vi "CRYChange post_xyz mode.vi"(6 "Wave In":T2={"Waveform"={"X0"=0.0, "dX"=0.0, "Y"=[]}, "X data"=1, "Y data"=0, "Y axis"=0, "X unit"="s", "Y unit"="", "Y dB ref"=1.0, "display Y"=TRUE, "display X"=FALSE, "Overload?"=FALSE, "Test Info"="", "Step No."=0, "Name"="", "protected"=FALSE, "Sqc history"=[], "Signal Channel ID"=0, "Plot Settings"={"Color"=0, "Interpolation"=0, "Point Style"=0, "Line Style"=0, "Point Color"=0, "Line Width"=0, "Bar Plot Style"=0, "Fill To"=0}, "AutoProtect"=FALSE} {"Y dB ref" format="%.1f"; "Y axis" items=["Log", "Lin"]; "Y data" items=["dB", "Lin"]; "X data" items=["dB", "Lin"]}, 7 "Work in":u16(slide), 8 "Value In":T1={"Name"="", "Curve"=[], "X data"=1, "Y data"=1, "Z data"=1, "X axis"=0, "Y axis"=1, "Z axis"=1, "X unit"="Hz", "Y unit"="", "Z unit"="deg.", "X dB ref"=1.0, "Y dB ref"=1.0, "Z dB ref"=1.0, "single val"=FALSE, "protected"=FALSE, "display X"=TRUE, "display Y"=TRUE, "display Z"=TRUE, "Test Info"="", "Step No."=0, "Plot Settings"={"Color"=0, "Interpolation"=0, "Point Style"=0, "Line Style"=0, "Point Color"=0, "Line Width"=0, "Bar Plot Style"=0, "Fill To"=0}, "AutoProtect"=FALSE} {"Z data" items=["dB", "Lin"]; "X data" items=["dB", "Lin"]; "Y data" items=["dB", "Lin"]; "Z dB ref" format="%.1f"; "Z axis" items=["Log", "Lin"]; "X dB ref" format="%.1f"; "X axis" items=["Log", "Lin"]; "Y axis" items=["Log", "Lin"]; "Y dB ref" format="%.1f"; "Curve"."z" format="%.2f"; "Curve"."y" format="%.2f"; "Curve"."x" format="%.2f"}, 9 "Curve In":T1={"Name"="", "Curve"=[], "X data"=1, "Y data"=1, "Z data"=1, "X axis"=0, "Y axis"=1, "Z axis"=1, "X unit"="Hz", "Y unit"="", "Z unit"="deg.", "X dB ref"=1.0, "Y dB ref"=1.0, "Z dB ref"=1.0, "single val"=FALSE, "protected"=FALSE, "display X"=TRUE, "display Y"=TRUE, "display Z"=TRUE, "Test Info"="", "Step No."=0, "Plot Settings"={"Color"=0, "Interpolation"=0, "Point Style"=0, "Line Style"=0, "Point Color"=0, "Line Width"=0, "Bar Plot Style"=0, "Fill To"=0}, "AutoProtect"=FALSE} {"Z data" items=["dB", "Lin"]; "X data" items=["dB", "Lin"]; "Y data" items=["dB", "Lin"]; "Z dB ref" format="%.1f"; "Z axis" items=["Log", "Lin"]; "X dB ref" format="%.1f"; "X axis" items=["Log", "Lin"]; "Y axis" items=["Log", "Lin"]; "Y dB ref" format="%.1f"; "Curve"."z" format="%.2f"; "Curve"."y" format="%.2f"; "Curve"."x" format="%.2f"}, 10 "XYZ Mode In":u16=1, 11 "Type In":enum16{"Curves", "Values", "Results", "WFM"}(ring)) -> (0 "Value":dbl, 1 "Tip Out":string, 2 "Unit Out":string, 3 "Value Out":string, 4 "Is Val&log":u16)   [LabVIEW 2013]
uses:
  Typedef Control/CRYWaveform Cluster.ctl
  Typedef Control/CRYData Cluster.ctl
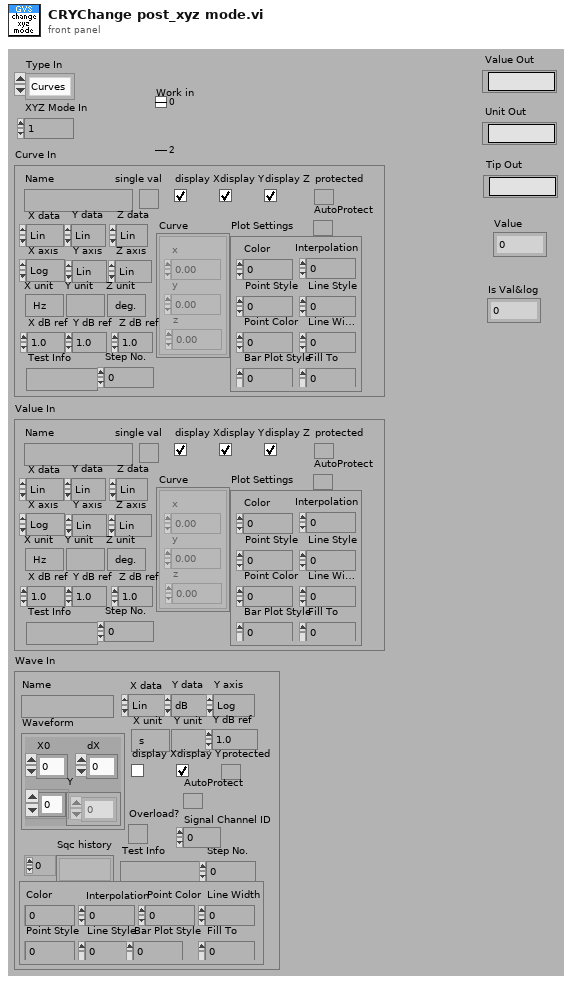
[diagram p1: front panel]
types:
  T1 = typedef "CRYData Cluster.ctl" = cluster{"Name":string, "Curve":cluster{"x":dbl, "y":dbl, "z":dbl}[], "X data":u16, "Y data":u16, "Z data":u16, "X axis":u16, "Y axis":u16, "Z axis":u16, "X unit":string, "Y unit":string, "Z unit":string, "X dB ref":dbl, "Y dB ref":dbl, "Z dB ref":dbl, "single val":bool, "protected":bool, "display X":bool, "display Y":bool, "display Z":bool, "Test Info":string, "Step No.":i32, "Plot Settings":cluster{"Color":u32, "Interpolation":u8, "Point Style":u8, "Line Style":u8, "Point Color":u32, "Line Width":u8, "Bar Plot Style":u8, "Fill To":i16}, "AutoProtect":bool}
  T2 = typedef "CRYWaveform Cluster.ctl" = cluster{"Waveform":cluster{"X0":dbl, "dX":dbl, "Y":sgl[]}, "X data":u16, "Y data":u16, "Y axis":u16, "X unit":string, "Y unit":string, "Y dB ref":dbl, "display Y":bool, "display X":bool, "Overload?":bool, "Test Info":string, "Step No.":i32, "Name":string, "protected":bool, "Sqc history":string[], "Signal Channel ID":i32, "Plot Settings":cluster{"Color":u32, "Interpolation":u8, "Point Style":u8, "Line Style":u8, "Point Color":u32, "Line Width":u8, "Bar Plot Style":u8, "Fill To":i16}, "AutoProtect":bool}
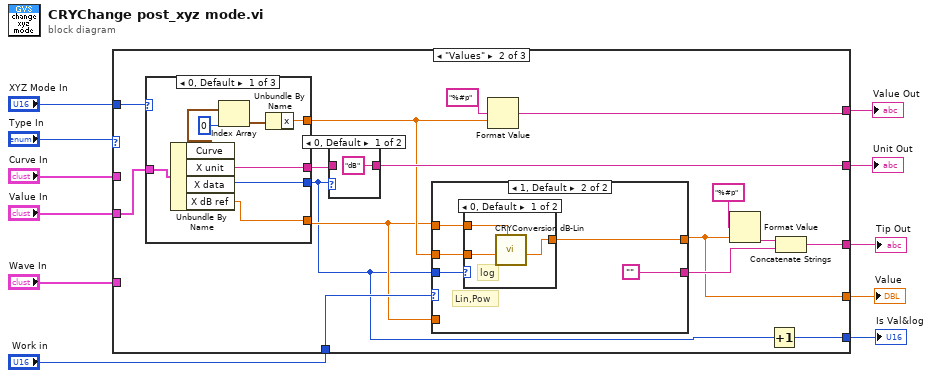
[diagram p0: block diagram]
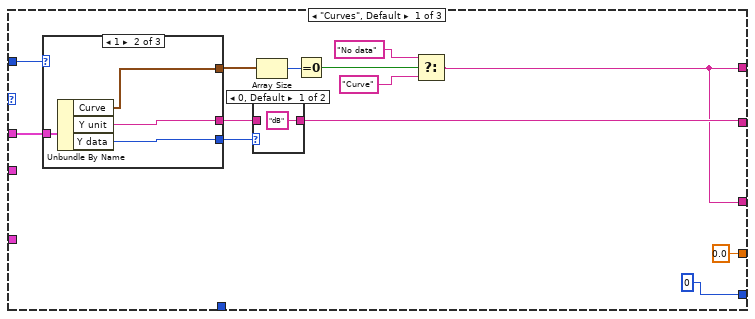
[diagram p2: hidden frame]
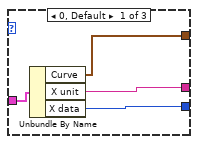
[diagram p4: hidden frame]
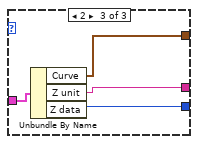
[diagram p5: hidden frame]
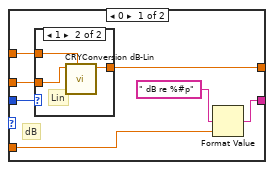
[diagram p7: hidden frame]
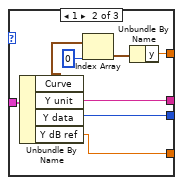
[diagram p10: hidden frame]
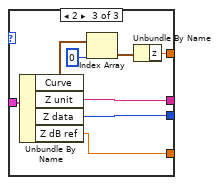
[diagram p11: hidden frame]
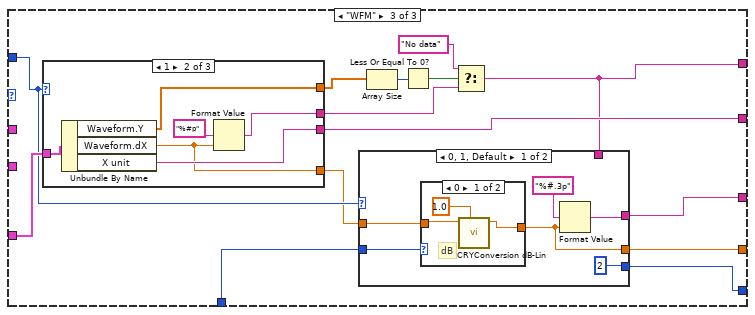
[diagram p12: hidden frame]
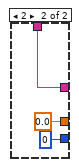
[diagram p14: hidden frame]
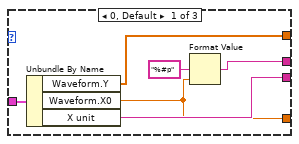
[diagram p15: hidden frame]
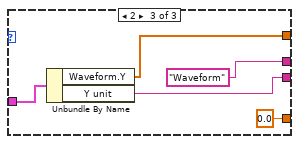
[diagram p16: hidden frame]
diagram:
  n1 = case shown="\"Values\"" "Type In" {
    tunnel: [w20 w48 w114] -> w11
    tunnel: "XYZ Mode In" -> [w24 w54 w107]
    tunnel: "Curve In" -> [w23 _ _]
    tunnel: "Value In" -> [_ w53 _]
    tunnel: "Wave In" -> [_ _ w113]
    tunnel: [w14 w51 w103] -> w4
    tunnel: "Work in" -> [_ w50 w106]
    tunnel: [w14 w44 w104] -> w3
    tunnel: [0.0 ("dX") w41 w102] -> w2
    tunnel: [0 w39 w101] -> w1
    frame "Curves", Default {
      n2 = case shown="1" w24 {
        tunnel: w23 -> [w30 w34 w38]
        tunnel: [w29 w33 w37] -> w21
        tunnel: [w28 w32 w36] -> w22
        tunnel: [w27 w31 w35] -> w18
        frame 0, Default {
          n3 = Unbundle By Name(w30) -> ("Curve"=w27:cluster{"x":dbl, "y":dbl, "z":dbl}[], "X unit"=w29:string, "X data"=w28:u16)
        }
        frame 1 {
          n4 = Unbundle By Name(w34) -> ("Curve"=w31:cluster{"x":dbl, "y":dbl, "z":dbl}[], "Y unit"=w33:string, "Y data"=w32:u16)
        }
        frame 2 {
          n5 = Unbundle By Name(w38) -> ("Curve"=w35:cluster{"x":dbl, "y":dbl, "z":dbl}[], "Z unit"=w37:string, "Z data"=w36:u16)
        }
      }
      n6 = case shown="0, Default" w22 {
        tunnel: w21 -> [_ w26]
        tunnel: ["dB" ("Y unit") w26] -> w20
        frame 0, Default {
        }
        frame 1 {
        }
      }
      n7 = Array Size(array=w18) -> (size(s)=w19:i32)
      n8 = Equal To 0?(x=w19) -> (x = 0?=w15:bool)
      n9 = Select(t="No data" ("f"), s=w15, f="Curve") -> (s? t:f=w14:string)
    }
    frame "Values" {
      n10 = case shown="0, Default" w54 {
        tunnel: w53 -> [w84 w89 w97]
        tunnel: [w80 w88 w96] -> w47
        tunnel: [w79 w87 w95] -> w49
        tunnel: [w78 w86 w94] -> w40
        tunnel: [w77 w85 w93] -> w43
        frame 0, Default {
          n11 = Unbundle By Name(w84) -> ("Curve"=w83:cluster{"x":dbl, "y":dbl, "z":dbl}[], "X unit"=w79:string, "X data"=w78:u16, "X dB ref"=w77:dbl)
          n12 = Index Array(array=w83, index=0) -> (element=w81:cluster{"x":dbl, "y":dbl, "z":dbl})
          n13 = Unbundle By Name(w81) -> ("x"=w80:dbl)
        }
        frame 1 {
          n14 = Unbundle By Name(w89) -> ("Curve"=w90:cluster{"x":dbl, "y":dbl, "z":dbl}[], "Y unit"=w87:string, "Y data"=w86:u16, "Y dB ref"=w85:dbl)
          n15 = Index Array(array=w90, index=0) -> (element=w92:cluster{"x":dbl, "y":dbl, "z":dbl})
          n16 = Unbundle By Name(w92) -> ("y"=w88:dbl)
        }
        frame 2 {
          n17 = Unbundle By Name(w97) -> ("Curve"=w98:cluster{"x":dbl, "y":dbl, "z":dbl}[], "Z unit"=w95:string, "Z data"=w94:u16, "Z dB ref"=w93:dbl)
          n18 = Index Array(array=w98, index=0) -> (element=w100:cluster{"x":dbl, "y":dbl, "z":dbl})
          n19 = Unbundle By Name(w100) -> ("z"=w96:dbl)
        }
      }
      n20 = case shown="0, Default" w40 {
        tunnel: w49 -> [_ w56]
        tunnel: ["dB" ("Y unit") w56] -> w48
        frame 0, Default {
        }
        frame 1 {
        }
      }
      n21 = case shown="1, Default" w50 {
        tunnel: w40 -> [w60 w69]
        tunnel: w47 -> [w63 w72]
        tunnel: w43 -> [w61 w70]
        tunnel: [w62 w71] -> w41
        tunnel: w43 -> [w58 _]
        tunnel: [w57 ""] -> w42
        frame 0 {
          # "dB"
          n22 = case shown="1" w60 {
            tunnel: w63 -> [w64 w66]
            tunnel: w61 -> [_ w67]
            tunnel: [w64 w65] -> w62
            frame 0, Default {
              # "log"
            }
            frame 1 {
              # "Lin"
              n23 = call "CRYConversion dB-Lin.vi"("dB ref."=w67, "Lin In"=w66) -> ("Log Out"=w65:dbl)  [unwired: 4 in, 3 out]
            }
          }
          n24 = Format Value(format string=" dB re %#p", value (0)=w58) -> (output string=w57:string)  [unwired: 1 in]
        }
        frame 1, Default {
          # "Lin,Pow"
          n25 = case shown="0, Default" w69 {
            tunnel: w72 -> [w75 w76]
            tunnel: w70 -> [w73 _]
            tunnel: [w74 w76] -> w71
            frame 0, Default {
              # "log"
              n26 = call "CRYConversion dB-Lin.vi"("dB ref."=w73, "Log In"=w75) -> ("Lin Out"=w74:dbl)  [unwired: 4 in, 3 out]
            }
            frame 1 {
              # "Lin"
            }
          }
        }
      }
      n27 = Format Value(format string="%#p", value (0)=w47) -> (output string=w51:string)  [unwired: 1 in]
      n28 = Format Value(format string="%#p", value (0)=w41) -> (output string=w45:string)  [unwired: 1 in]
      n29 = Increment(x=w40) -> (x+1=w39:u16)
      n30 = Concatenate Strings(w45, w42) -> (w44:string)
    }
    frame "WFM" {
      n31 = case shown="1" w107 {
        tunnel: w113 -> [w133 w139 w144]
        tunnel: [w132 w138 w143] -> w114
        tunnel: [w130 w136 "Waveform" ("output string")] -> w108
        tunnel: [w129 w135 w141] -> w109
        tunnel: [w128 w134 0.0 ("dX")] -> w105
        frame 0, Default {
          n32 = Unbundle By Name(w133) -> ("Waveform.Y"=w129:sgl[], "Waveform.X0"=w128:dbl, "X unit"=w132:string)
          n33 = Format Value(format string="%#p", value (0)=w128) -> (output string=w130:string)  [unwired: 1 in]
        }
        frame 1 {
          n34 = Unbundle By Name(w139) -> ("Waveform.Y"=w135:sgl[], "Waveform.dX"=w134:dbl, "X unit"=w138:string)
          n35 = Format Value(format string="%#p", value (0)=w134) -> (output string=w136:string)  [unwired: 1 in]
        }
        frame 2 {
          n36 = Unbundle By Name(w144) -> ("Waveform.Y"=w141:sgl[], "Y unit"=w143:string)
        }
      }
      n37 = Array Size(array=w109) -> (size(s)=w111:i32)
      n38 = Less Or Equal To 0?(x=w111) -> (x <= 0?=w110:bool)
      n39 = Select(t="No data" ("f"), s=w110, f=w108) -> (s? t:f=w103:string)
      n40 = case shown="0, 1, Default" w107 {
        tunnel: w106 -> [w119 _]
        tunnel: w105 -> [w118 _]
        tunnel: [w117 w127] -> w104
        tunnel: w103 -> [_ w127]
        tunnel: [w116 0.0 ("dX")] -> w102
        tunnel: [2 0] -> w101
        frame 0, 1, Default {
          n41 = case shown="0" w119 {
            tunnel: [w121 w124] -> w116
            tunnel: w118 -> [w123 w124]
            frame 0 {
              # "dB"
              n42 = call "CRYConversion dB-Lin.vi"("dB ref."=1.0, "Lin In"=w123) -> ("Log Out"=w121:dbl)  [unwired: 4 in, 3 out]
            }
            frame 1, Default {
              # "Lin,Pow"
            }
          }
          n43 = Format Value(format string="%#.3p", value (0)=w116) -> (output string=w117:string)  [unwired: 1 in]
        }
        frame 2 {
        }
      }
    }
  }
  "Value Out" <- w4
  "Unit Out" <- w11
  "Tip Out" <- w3
  "Value" <- w2
  "Is Val&log" <- w1
